vi "호출자(엄격).vi"() -> ()   [LabVIEW 2014]
uses:
  <vilib>/measure/maspectr.llb/Power Spectrum and PSD Export Mode.ctl
  <vilib>/Analysis/4window.llb/windowTd.ctl
  <vilib>/measure/NI_MAPro.lvlib
  <vilib>/Analysis/NI_AALPro.lvlib
panel:
  out "웨이브폼 그래프":cluster{"f0":dbl, "df":dbl, "magnitude":dbl[]}
  in  "dB On (F)":bool
  in  "window":T1 items=["사각형"=0, "해닝"=1, "해밍"=2, "블랙맨-해리스"=3, "정밀한 블랙맨"=4, "블랙맨"=5, "플랫 탑(Flat Top)"=6, "4항 블랙맨-해리스 "=7, "7항 블랙맨-해리스"=8, "낮은 사이드로브"=9, "블랙맨 누탈"=11, "삼각파"=30, "바틀렛-해닝"=31, "보먼"=32, "파젠"=33, "웰치"=34, "카이저"=60, "돌프-체비셰프"=61, "가우스"=62]
  in  "export mode":T2 items=["파워 스펙트럼", "파워 스펙트럼 밀도"]
  in  "frequency":dbl
  in  "signal type":T3(ring)
  out "에러 출력":errorcluster
  in  "vi 경로":path
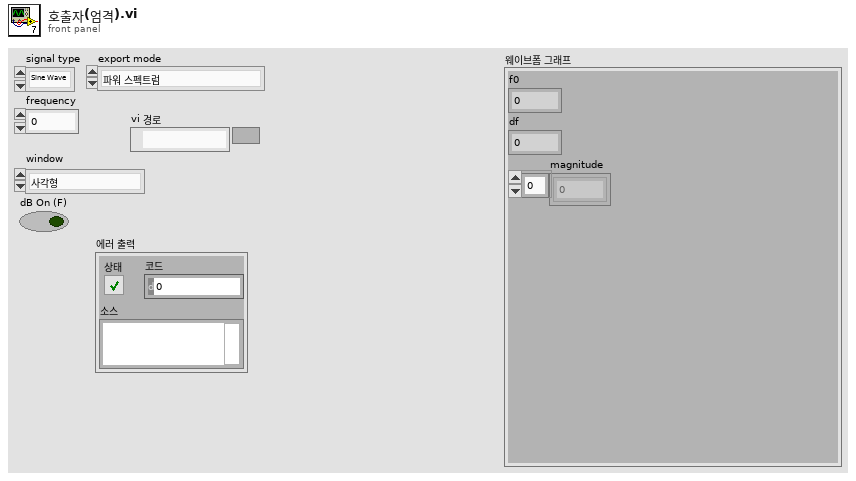
[diagram p1: front panel]
types:
  T1 = typedef "NI_AALPro.lvlib/windowTd.ctl" = u32
  T2 = typedef "NI_MAPro.lvlib/Power Spectrum and PSD Export Mode.ctl" = u16
  T3 = enum16{"Sine Wave", "Triangle Wave", "Square Wave", "Sawtooth Wave"}
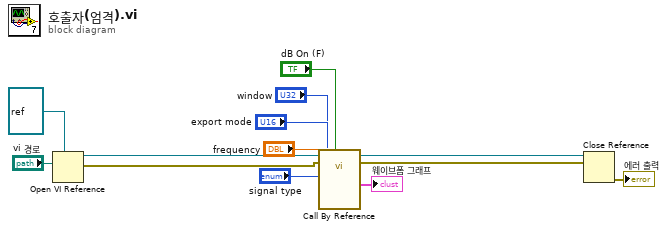
[diagram p0: block diagram]
diagram:
  n1 = Open VI Reference(type specifier VI Refnum (for type only)=refnum<vi> refnum ("타입 지정자 VI 참조 번호(타입만)"), vi path="vi 경로") -> (vi reference=w7:refnum<vi>, error out=w11:errorcluster)  [unwired: 4 in]
  n2 = call-by-ref "?"(reference=w7, error in=w11, "dB On (F)"="dB On (F)", "window"="window", "export mode"="export mode", "frequency"="frequency", "signal type"="signal type") -> (reference out=w13:refnum<vi>, error out=w10:errorcluster, "웨이브폼 그래프"=→"웨이브폼 그래프":cluster{"f0":dbl, "df":dbl, "magnitude":dbl[]})  [unwired: 6 in]
  n3 = Close Reference(reference=w13, error in (no error)=w10) -> (error out=→"에러 출력":errorcluster)
